vi "Set reporter if null.vi"(10 "results reporter":refnum<class "results reporter.lvclass">, 11 "task in":refnum<class "task.lvclass">) -> (3 "task out":refnum<class "task.lvclass">)   [LabVIEW 2013, in "task.lvclass"]
uses:
  task.lvclass
  results reporter/results reporter.lvclass
  task.lvclass/task.ctl
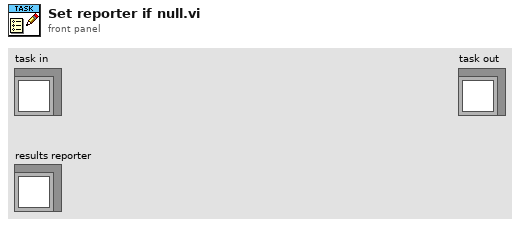
[diagram p1: front panel]
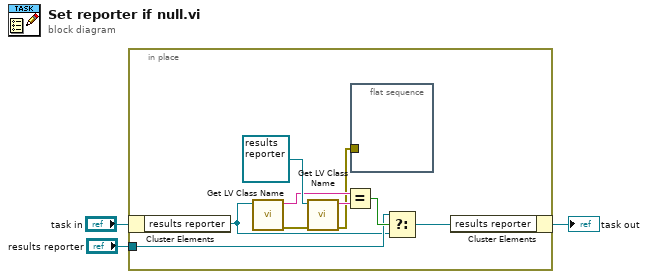
[diagram p0: block diagram]
diagram:
  n1 = in-place {
    in-place-border: "results reporter" -> [w6]
    n2 = in-place-cluster #1("task in") -> ("results reporter"=w5:refnum<class "results reporter.lvclass">)
    n3 = call <vilib>:"Get LV Class Name.vi"("object"=w5) -> ("error out"=w11:errorcluster, "class name"=w9:string)  [unwired: 9 in]
    n4 = call <vilib>:"Get LV Class Name.vi"("error in (no error)"=w11, "object"=refnum<class "results reporter.lvclass"> refnum ("results reporter")) -> ("error out"=w8:errorcluster, "class name"=w10:string)  [unwired: 8 in]
    n5 = Equal?(x=w9, y=w10) -> (x = y?=w7:bool)
    n6 = flat-sequence {
      tunnel: w8 -> [_]
      frame #0 {
      }
    }
    n7 = Select(t=w6, s=w7, f=w5) -> (s? t:f=w4:refnum<class "results reporter.lvclass">)
    n8 = in-place-cluster #1("results reporter"=w4) -> (→"task out":refnum<class "task.lvclass">)
  }
